vi "Open.vi"(8 "error in (no error)":errorcluster, 11 "MelsecTCP in":refnum<class "MelsecMcNet.lvclass">) -> (0 "error out":errorcluster, 2 "IsSuccess":bool, 3 "MelsecTCP out":refnum<class "MelsecMcNet.lvclass">)   [LabVIEW 2020, in "MelsecMcNet.lvclass"]
uses:
  MelsecMcNet.lvclass
  C:/Users/Fred Guo/Desktop/API_Salcomp_CMES/Libraries/HslCommunication/HslCommunication.dll
  HslCommunication.dll
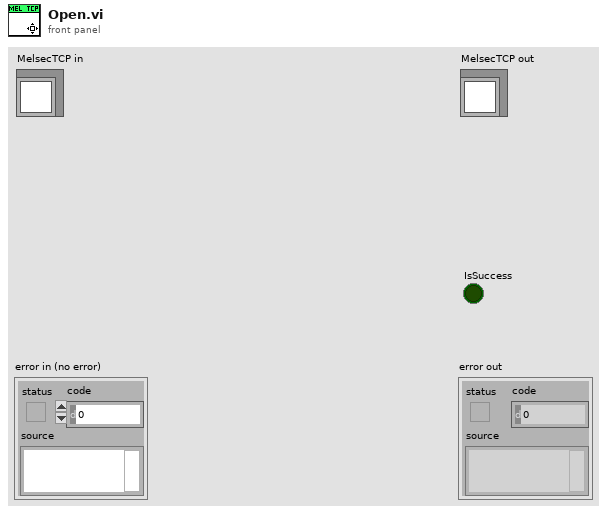
[diagram p1: front panel]
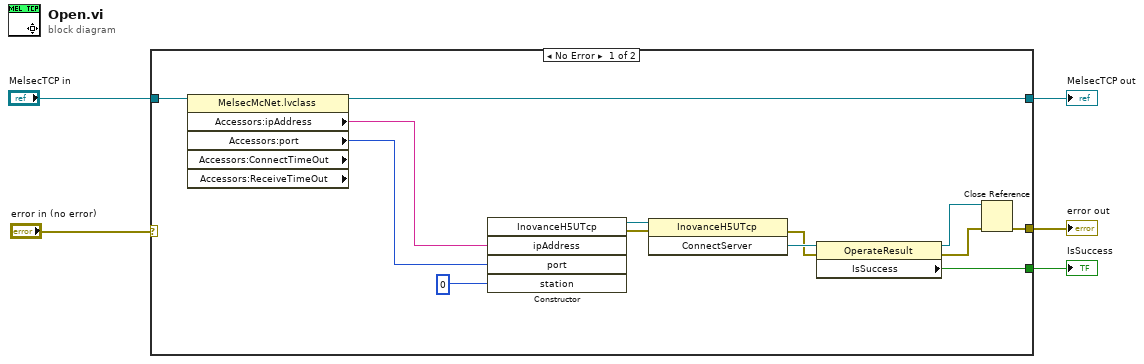
[diagram p0: block diagram]
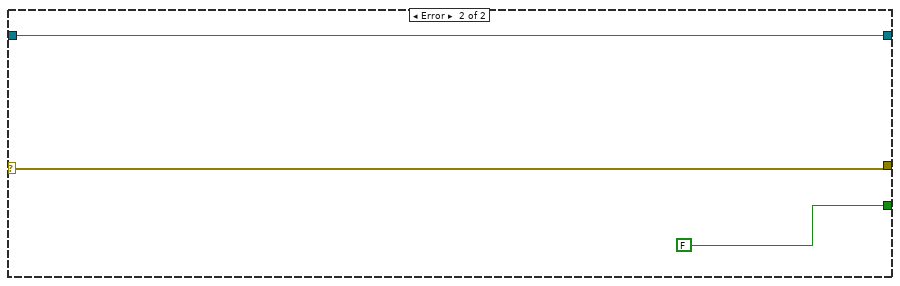
[diagram p2: hidden frame]
diagram:
  n1 = case shown="No Error" "error in (no error)" {
    selector: "error in (no error)" -> [_ w21]
    tunnel: "MelsecTCP in" -> [w18 w20]
    tunnel: [w13 w21] -> w4
    tunnel: [w12 w20] -> w2
    tunnel: [w11 FALSE ("IsSuccess")] -> w1
    frame No Error {
      n2 = property class="MelsecMcNet.lvclass" props=["Accessors:ipAddress", "Accessors:port", "Accessors:ConnectTimeOut", "Accessors:ReceiveTimeOut"](reference=w18) -> (reference out=w12:refnum<class "MelsecMcNet.lvclass">, "Accessors:ipAddress"=w10:string, "Accessors:port"=w9:i32)  [unwired: 1 in, 3 out]
      n3 = constructor class="InovanceH5UTcp"("ipAddress"=w10, "port"=w9, "station"=u8 0) -> (reference out=w8:refnum<k24>, error out=w7:errorcluster)  [unwired: 3 in, 4 out]
      n4 = invoke class="InovanceH5UTcp" method="ConnectServer"(reference=w8, error in=w7) -> (error out=w15:errorcluster, "ConnectServer"=w17:refnum<k24>)  [unwired: 1 in, 1 out]
      n5 = property class="OperateResult"(reference=w17, error in=w15) -> (reference out=w16:refnum<k24>, error out=w14:errorcluster, "IsSuccess"=w11:bool)
      n6 = Close Reference(reference=w16, error in (no error)=w14) -> (error out=w13:errorcluster)
    }
    frame Error {
    }
  }
  "error out" <- w4
  "MelsecTCP out" <- w2
  "IsSuccess" <- w1
